vi "HEUI_LEDs to Actual LEDs.vi"(7 "HEUI_LEDs":T1) -> (8 "Actual LEDs":bool[](array[boolean]))   [LabVIEW 2016, in "2015 VA Washer.lvlib"]
uses:
  Projects/2015 VA Washer.lvlib
  controls/HEUI_LEDs.ctl
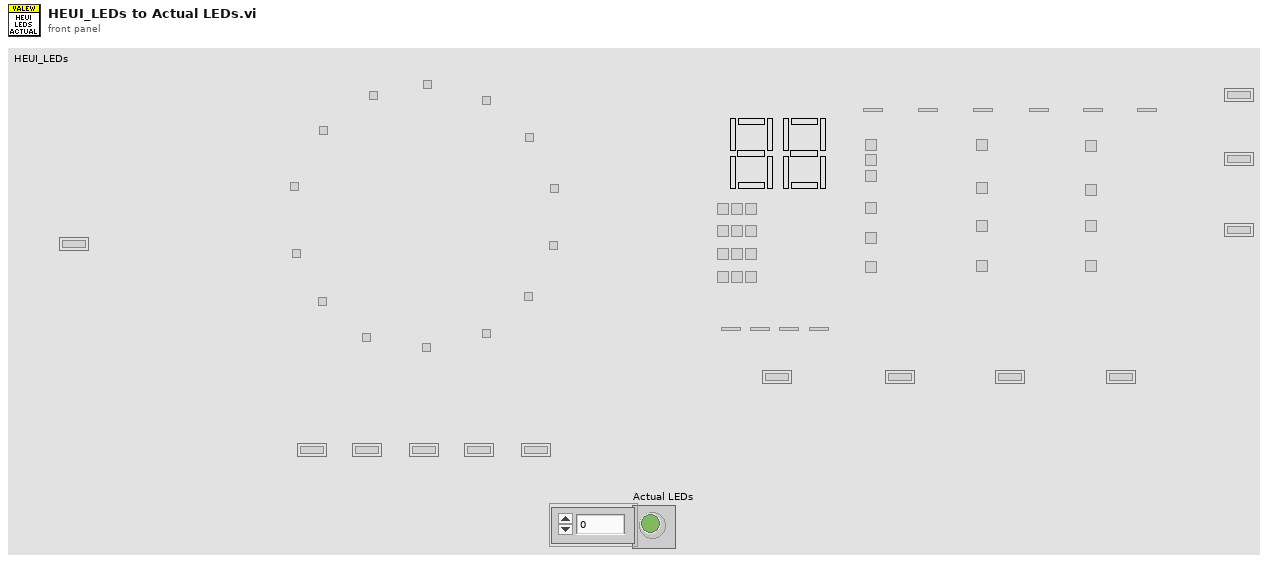
[diagram p1: front panel]
types:
  T1 = typedef "2015 VA Washer.lvlib/HEUI_LEDs.ctl" = cluster{"Z101 - Start":bool, "Z103 - Colors":bool, "Z104 - Whites":bool, "Z105 - Towels":bool, "Z106 - Bulky Items":bool, "Z107 - Heavy Duty":bool, "Z108 - Jeans":bool, "Z109 - Basket Clean":bool, "Z110 - Drain and Spin":bool, "Z111 - Rinse and Spin":bool, "Z112 - Speed Wash":bool, "Z113 - Active Wear":bool, "Z114 - Hand Wash":bool, "Z115 - Delicates":bool, "Z116 - Easy Care":bool, "Z117 - Tomato":bool, "Z118 - Wine":bool, "Z119 - Blood":bool, "Z120 - Grass":bool, "Z121 - Dirt":bool, "Z122_MSB_A":bool, "Z123_MSB_B":bool, "Z124_MSB_G":bool, "Z125_MSB_C":bool, "Z126_MSB_D":bool, "Z127_MSB_E":bool, "Z128_MSB_F":bool, "Z129_LSB_A":bool, "Z130_LSB_B":bool, "Z131_LSB_G":bool, "Z132_LSB_C":bool, "Z133_LSB_D":bool, "Z134_LSB_E":bool, "Z135_LSB_F":bool, "Z136 - Pause":bool, "Z137 - Pause":bool, "Z138 - Lock Controls":bool, "Z139 - Lock Controls":bool, "Z140 - Lock Controls":bool, "Z141 - Lid Lock":bool, "Z142 - Lid Lock":bool, "Z143 - Lid Lock":bool, "Z144 - Good":bool, "Z145":bool, "Z146":bool, "Z147 - Better":bool, "Z148 - Delay":bool, "Z149 - Fill":bool, "Z150 - Soak":bool, "Z151 - Wash":bool, "Z152 - Rinse":bool, "Z153 - Spin":bool, "Z154 - Hot":bool, "Z155 - Warm":bool, "Z156 - Colors":bool, "Z157 - Cool":bool, "Z158 - Cold":bool, "Z159 - Tap Cold":bool, "Z160 - Extra Heavy":bool, "Z161 - Heavy":bool, "Z162 - Normal":bool, "Z163 - Light":bool, "Z164 - Max Spin":bool, "Z165 - More Spin":bool, "Z166 - Normal Spin":bool, "Z167 - No Spin":bool, "Z168 - Extra Rinse":bool, "Z170 - Deep Rinse":bool, "Z171 - Auto Soak":bool, "Z172 - Warm Rinse":bool, "Z173 - Deep Fill":bool, "Z174 - My Cycles":bool, "Z175 - Delay Wash":bool, "Z176 - Spin Stop":bool, "Z177 - Spin Stop":bool, "Z178 - Spin Stop":bool, "Z179 - Pause":bool, "Z109":bool, "Z110":bool, "Z123":bool, "Z124":bool, "Z140":bool, "Unused0":bool, "Unused1":bool, "Unused2":bool, "Unused3":bool, "Channel_Off":bool, "Channel_Cycle_Unmapped":bool}
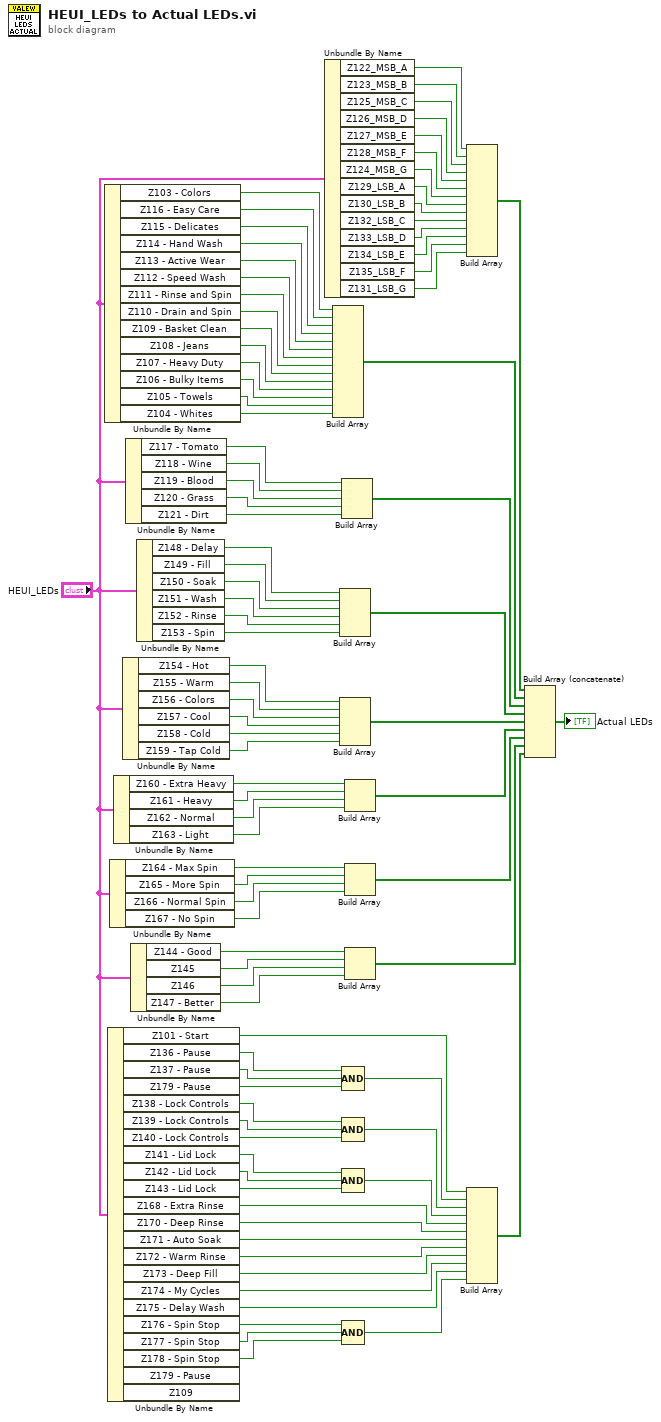
[diagram p0: block diagram]
diagram:
  n1 = Unbundle By Name("HEUI_LEDs") -> ("Z103 - Colors"=w77:bool, "Z116 - Easy Care"=w76:bool, "Z115 - Delicates"=w75:bool, "Z114 - Hand Wash"=w74:bool, "Z113 - Active Wear"=w73:bool, "Z112 - Speed Wash"=w72:bool, "Z111 - Rinse and Spin"=w71:bool, "Z110 - Drain and Spin"=w70:bool, "Z109 - Basket Clean"=w69:bool, "Z108 - Jeans"=w68:bool, "Z107 - Heavy Duty"=w67:bool, "Z106 - Bulky Items"=w66:bool, "Z105 - Towels"=w65:bool, "Z104 - Whites"=w63:bool)
  n2 = Unbundle By Name("HEUI_LEDs") -> ("Z101 - Start"=w17:bool, "Z136 - Pause"=w26:bool, "Z137 - Pause"=w25:bool, "Z179 - Pause"=w24:bool, "Z138 - Lock Controls"=w23:bool, "Z139 - Lock Controls"=w22:bool, "Z140 - Lock Controls"=w21:bool, "Z141 - Lid Lock"=w20:bool, "Z142 - Lid Lock"=w19:bool, "Z143 - Lid Lock"=w18:bool, "Z168 - Extra Rinse"=w13:bool, "Z170 - Deep Rinse"=w12:bool, "Z171 - Auto Soak"=w11:bool, "Z172 - Warm Rinse"=w10:bool, "Z173 - Deep Fill"=w9:bool, "Z174 - My Cycles"=w8:bool, "Z175 - Delay Wash"=w7:bool, "Z176 - Spin Stop"=w6:bool, "Z177 - Spin Stop"=w5:bool, "Z178 - Spin Stop"=w4:bool)  [unwired: 2 out]
  n3 = Unbundle By Name("HEUI_LEDs") -> ("Z164 - Max Spin"=w37:bool, "Z165 - More Spin"=w36:bool, "Z166 - Normal Spin"=w35:bool, "Z167 - No Spin"=w34:bool)
  n4 = Unbundle By Name("HEUI_LEDs") -> ("Z160 - Extra Heavy"=w42:bool, "Z161 - Heavy"=w41:bool, "Z162 - Normal"=w40:bool, "Z163 - Light"=w39:bool)
  n5 = Unbundle By Name("HEUI_LEDs") -> ("Z154 - Hot"=w49:bool, "Z155 - Warm"=w48:bool, "Z156 - Colors"=w47:bool, "Z157 - Cool"=w46:bool, "Z158 - Cold"=w45:bool, "Z159 - Tap Cold"=w44:bool)
  n6 = Unbundle By Name("HEUI_LEDs") -> ("Z117 - Tomato"=w62:bool, "Z118 - Wine"=w61:bool, "Z119 - Blood"=w60:bool, "Z120 - Grass"=w59:bool, "Z121 - Dirt"=w58:bool)
  n7 = Unbundle By Name("HEUI_LEDs") -> ("Z144 - Good"=w32:bool, "Z145"=w31:bool, "Z146"=w30:bool, "Z147 - Better"=w29:bool)
  n8 = Unbundle By Name("HEUI_LEDs") -> ("Z148 - Delay"=w56:bool, "Z149 - Fill"=w55:bool, "Z150 - Soak"=w54:bool, "Z151 - Wash"=w53:bool, "Z152 - Rinse"=w52:bool, "Z153 - Spin"=w51:bool)
  n9 = Unbundle By Name("HEUI_LEDs") -> ("Z122_MSB_A"=w92:bool, "Z123_MSB_B"=w91:bool, "Z125_MSB_C"=w90:bool, "Z126_MSB_D"=w89:bool, "Z127_MSB_E"=w88:bool, "Z128_MSB_F"=w87:bool, "Z124_MSB_G"=w86:bool, "Z129_LSB_A"=w85:bool, "Z130_LSB_B"=w84:bool, "Z132_LSB_C"=w83:bool, "Z133_LSB_D"=w82:bool, "Z134_LSB_E"=w81:bool, "Z135_LSB_F"=w80:bool, "Z131_LSB_G"=w79:bool)
  n10 = Build Array(w77, w76, w75, w74, w73, w72, w71, w70, w69, w68, w67, w66, w65, w63) -> (w64:bool[])
  n11 = Build Array(w56, w55, w54, w53, w52, w51) -> (w50:bool[])
  n12 = Build Array(w49, w48, w47, w46, w45, w44) -> (w43:bool[])
  n13 = Build Array(w62, w61, w60, w59, w58) -> (w57:bool[])
  n14 = Compound Arithmetic op=AND(w26, w25, w24) -> (w16:bool)
  n15 = Compound Arithmetic op=AND(w23, w22, w21) -> (w15:bool)
  n16 = Compound Arithmetic op=AND(w20, w19, w18) -> (w14:bool)
  n17 = Compound Arithmetic op=AND(w6, w5, w4) -> (w3:bool)
  n18 = Build Array(w42, w41, w40, w39) -> (w38:bool[])
  n19 = Build Array(w37, w36, w35, w34) -> (w33:bool[])
  n20 = Build Array(w32, w31, w30, w29) -> (w28:bool[])
  n21 = Build Array(w92, w91, w90, w89, w88, w87, w86, w85, w84, w83, w82, w81, w80, w79) -> (w78:bool[])
  n22 = Build Array(w17, w16, w15, w14, w13, w12, w11, w10, w9, w8, w7, w3) -> (w2:bool[])
  n23 = Build Array (concatenate)(w78, w64, w57, w50, w43, w38, w33, w28, w2) -> (→"Actual LEDs":bool[])
